vi "bpm.vi"() -> ()   [LabVIEW 2016]
doc: "The bpm vi uses the source rio to control the bpms on the high voltage deck. It can only work if the source rio is in the same project as this vi."
panel:
  in  "error in (no error)":errorcluster
  out "error out":errorcluster
  in  "stop":bool
  in  "Source 2 X10":bool
  in  "Source 2 BPM":bool
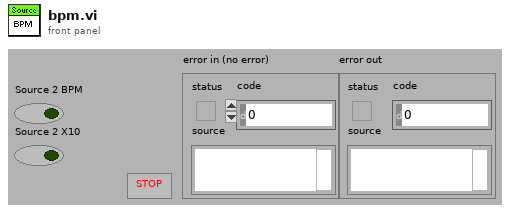
[diagram p1: front panel]
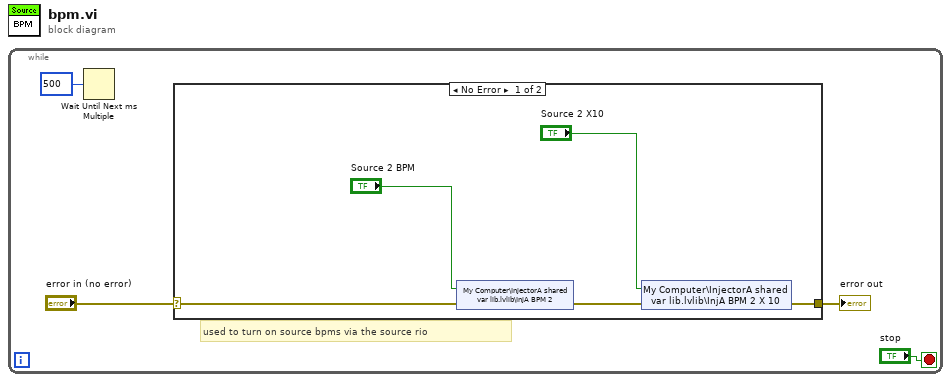
[diagram p0: block diagram]
diagram:
  n1 = while {
    stop <- "stop" stop-if-true
    # "used to turn on source bpms via the source rio"
    n2 = Wait Until Next ms Multiple(millisecond multiple=u32 500) -> ()  [unwired: 1 out]
    n3 = case shown="No Error" "error in (no error)" {
      selector: "error in (no error)" -> [w5 w10]
      tunnel: [w6 w10] -> w2
      frame No Error {
        n4 = shared-variable "My Computer\\InjectorA shared var lib.lvlib\\InjA BPM 2"("Source 2 BPM", error in=w5) -> (error out=w7:errorcluster)
        n5 = shared-variable "My Computer\\InjectorA shared var lib.lvlib\\InjA BPM 2 X 10"("Source 2 X10", error in=w7) -> (error out=w6:errorcluster)
      }
      frame Error {
      }
    }
    "error out" <- w2
  }
